vi "Get Time Profiler Data.vi"(8 "error in (no error)":errorcluster, 11 "Apriltag Detector in":refnum<class "AprilTag Detector.lvclass">) -> (0 "error out":errorcluster, 2 "Time Profile Entries":T1[](array[typedef]), 3 "Apriltag Detector":refnum<class "AprilTag Detector.lvclass">)   [LabVIEW 2020, in "feature_detection.lvlib" / "AprilTag Detector.lvclass"]
doc: "Detect the Tags in the Greyscale Image."
uses:
  AprilTag Detector.lvclass
  AprilTag Detector.lvclass/AprilTag Detector.ctl
  common/common.lvlib
  Time Profiler Entry.ctl
  common/bin/gartoolkit_fd_64-1.so
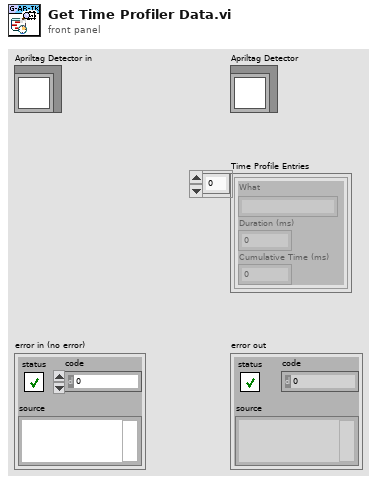
[diagram p1: front panel]
types:
  T1 = typedef "feature_detection.lvlib/AprilTag Detector.lvclass/Time Profiler Entry.ctl" = cluster{"What":string, "Duration (ms)":dbl, "Cumulative Time (ms)":dbl}
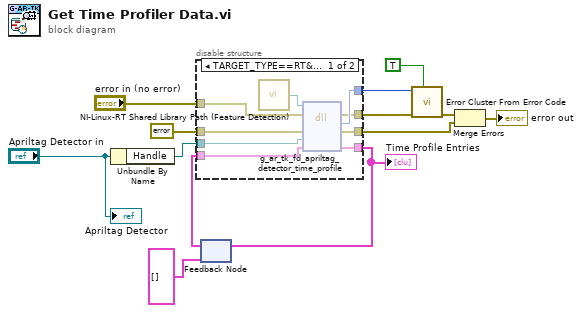
[diagram p0: block diagram]
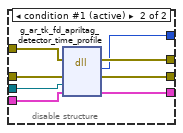
[diagram p2: hidden frame]
diagram:
  n1 = Unbundle By Name("Apriltag Detector in") -> ("Handle"=w8:refnum<data-value>)
  n2 = feedback #1(T1[] [] ("Array")) -> (w3:T1[])
  n3 = disable-structure shown="TARGET_TYPE==RT&&OS==Linux" {
    disable-tunnel: "error in (no error)" -> [w22 w30]
    disable-tunnel: errorcluster {"status"=FALSE, "code"=0, "source"=""} ("error constant") -> [w21 w29]
    disable-tunnel: w8 -> [w20 w28]
    disable-tunnel: w3 -> [w19 w27]
    disable-tunnel: [w15 w26] -> w7
    disable-tunnel: [w16 w25] -> w6
    disable-tunnel: [w17 w24] -> w5
    disable-tunnel: [w18 w23] -> w4
    frame condition #0 {
      n4 = call "NI-Linux-RT Shared Library Path (Feature Detection).vi"() -> ("Path"=w14:path)
      n5 = dll-call lib="home/john/g-augmented-reality-toolkit/LabVIEW/common/bin/gartoolkit_fd_*-1.*" fn="g_ar_tk_fd_apriltag_detector_time_profile" ("g_ar_toolkit.*.*:g_ar_tk_capture_context_create")(path in=w14, error in=w22, "error_cluster"=w21, "Detector_EDVR"=w20, "Time Profile Entries"=w19) -> (error out=w15:errorcluster, "return type"=w16:i32, "error_cluster"=w17:errorcluster, "Time Profile Entries"=w18:T1[])  [unwired: 2 in, 1 out]
    }
    frame condition #1 (active) {
      n6 = dll-call lib="home/john/g-augmented-reality-toolkit/LabVIEW/common/bin/gartoolkit_fd_*-1.*" fn="g_ar_tk_fd_apriltag_detector_time_profile" ("g_ar_toolkit.*.*:g_ar_tk_capture_context_create")(error in=w30, "error_cluster"=w29, "Detector_EDVR"=w28, "Time Profile Entries"=w27) -> (error out=w26:errorcluster, "return type"=w25:i32, "error_cluster"=w24:errorcluster, "Time Profile Entries"=w23:T1[])  [unwired: 3 in, 1 out]
    }
  }
  "Time Profile Entries" <- w4
  n7 = feedback-in #1(w4) -> ()
  n8 = call <vilib>:"Error Cluster From Error Code.vi"("show call chain? (False)"=TRUE, "error in (no error)"=w7, "error code (0)"=w6) -> ("error out"=w12:errorcluster)  [unwired: 6 in]
  n9 = Merge Errors(w12, w5) -> (→"error out":errorcluster)
  "Apriltag Detector" <- "Apriltag Detector in"
